vi "Set Personality with SN.vi"(8 "error in (no error)":errorcluster, 11 "roboRIO Connection Information":T1) -> (0 "error out":errorcluster)   [LabVIEW 2018, in "Personalities Tool.lvlib"]
doc: "This VI saves the RIO personality by the Serianl Number."
uses:
  Personalities Tool.lvlib
  Controls/roboRIO Connection Information.ctl
  Controls/Personality Type.ctl
  <vilib>/Utility/config.llb/Write Key (String).vi
  <vilib>/Utility/config.llb/NI_LVConfig.lvlib
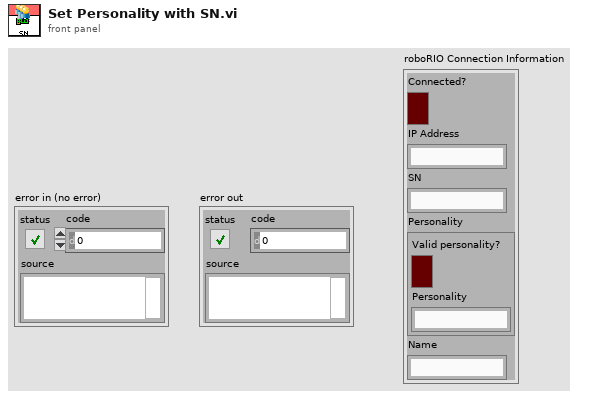
[diagram p1: front panel]
types:
  T1 = typedef "Personalities Tool.lvlib/roboRIO Connection Information.ctl" = cluster{"Connected?":bool, "IP Address":string, "SN":string, "Personality":T2, "Name":string}
  T2 = typedef "Personalities Tool.lvlib/Personality Type.ctl" = cluster{"Valid personality?":bool, "Personality":string}
  T3 = typedef "NI_LVConfig.lvlib/Config Data RefNum.ctl" = refnum<k1>
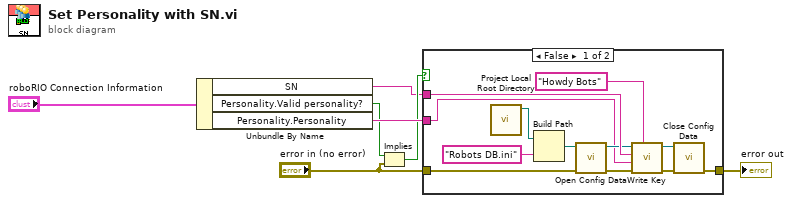
[diagram p0: block diagram]
diagram:
  n1 = Unbundle By Name("roboRIO Connection Information") -> ("SN"=w1:string, "Personality.Valid personality?"=w5:bool, "Personality.Personality"=w6:string)
  n2 = Implies(1:"error in (no error)", 2:w5) -> (0:w4:bool)
  n3 = case shown="False" w4 {
    tunnel: [w10 w20] -> w7
    tunnel: w1 -> [w19 _]
    tunnel: w6 -> [w9 _]
    tunnel: "error in (no error)" -> [w8 w20]
    frame False {
      n4 = call "Project Local Root Directory.vi"() -> ("Code root's folder"=w15:path)  [unwired: 11 in]
      n5 = Build Path(base path=w15, name or relative path="Robots DB.ini") -> (appended path=w16:path)
      n6 = call <vilib>:"Open Config Data.vi"("error in (no error)"=w8, "configuration file path"=w16) -> ("error out"=w12:errorcluster, "refnum"=w11:T3)  [unwired: 7 in, 1 out]
      n7 = call-poly <vilib>:"Write Key.vi"("section"="Howdy Bots", "error in (no error)"=w12, "value"=w9, "key"=w19, "refnum"=w11) -> ("error out"=w14:errorcluster, "refnum out"=w13:T3)  [unwired: 4 in, 1 out]
      n8 = call <vilib>:"Close Config Data.vi"("error in (no error)"=w14, "refnum"=w13) -> ("error out"=w10:errorcluster)  [unwired: 8 in, 1 out]
    }
    frame True {
    }
  }
  "error out" <- w7
